vi "Get value by Variant.vi"(8 "error in (no error)":errorcluster, 11 "Timestamp Column in":refnum<class "Timestamp Column.lvclass">) -> (0 "error out":errorcluster, 2 "Variant":variant, 3 "Timestamp Column out":refnum<class "Timestamp Column.lvclass">)   [LabVIEW 2020, in "Basic Columns.lvlib" / "Timestamp Column.lvclass"]
uses:
  Timestamp Column.lvclass
  Timestamp Column.lvclass/Timestamp Column.ctl
  Column Interface/Timestamp Rule Interface/Timestamp Rule Interface.lvclass
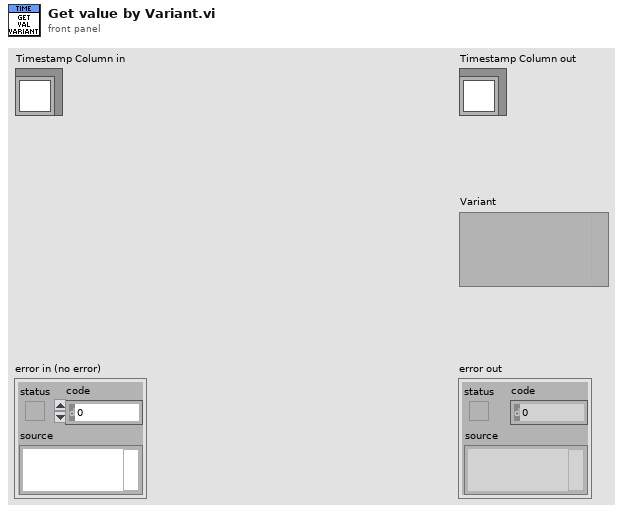
[diagram p1: front panel]
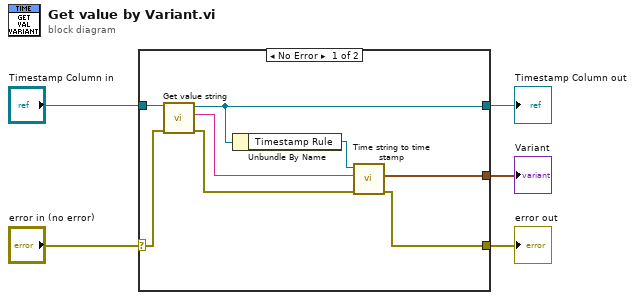
[diagram p0: block diagram]
diagram:
  n1 = case shown="No Error" "error in (no error)" {
    selector: "error in (no error)" -> [w7 w15]
    tunnel: [w8 w15] -> w4
    tunnel: "Timestamp Column in" -> [w13 w14]
    tunnel: [w12 w14] -> w2
    tunnel: [w6 _] -> w1
    frame No Error {
      n2 = call-dynamic "Get value string.vi"("error in (no error)"=w7, "Column in"=w13) -> ("error out"=w9:errorcluster, "Value"=w10:string, "Column out"=w12:refnum<class "Timestamp Column.lvclass">)  [unwired: 7 in]
      n3 = Unbundle By Name(w12) -> ("Timestamp Rule"=w11:refnum<class "Timestamp Rule Interface.lvclass">)
      n4 = call-dynamic "Time string to time stamp.vi"("error in (no error)"=w9, "Time String"=w10, "Timestamp Rule Interface in"=w11) -> ("error out"=w8:errorcluster, "Time Stamp"=w6:timestamp)  [unwired: 6 in, 1 out]
    }
    frame Error {
    }
  }
  "error out" <- w4
  "Timestamp Column out" <- w2
  "Variant" <- w1
